vi "get_double.vi"(8 "error in (no error)":errorcluster, 11 "TrajectoryTS090820Circular2D in":refnum<class "TrajectoryTS090820Circular2D.lvclass">) -> (0 "error out":errorcluster, 2 "double":bool, 3 "TrajectoryTS090820Circular2D out":refnum<class "TrajectoryTS090820Circular2D.lvclass">)   [LabVIEW 2010, in "TrajectoryTS090820Circular2D.lvclass"]
uses:
  TrajectoryTS090820Circular2D.lvclass
  TrajectoryTS090820Circular2D.lvclass/TrajectoryTS090820Circular2D.ctl
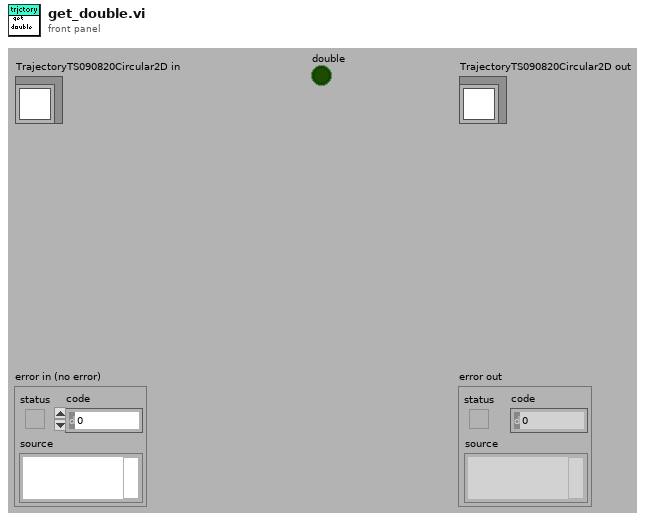
[diagram p1: front panel]
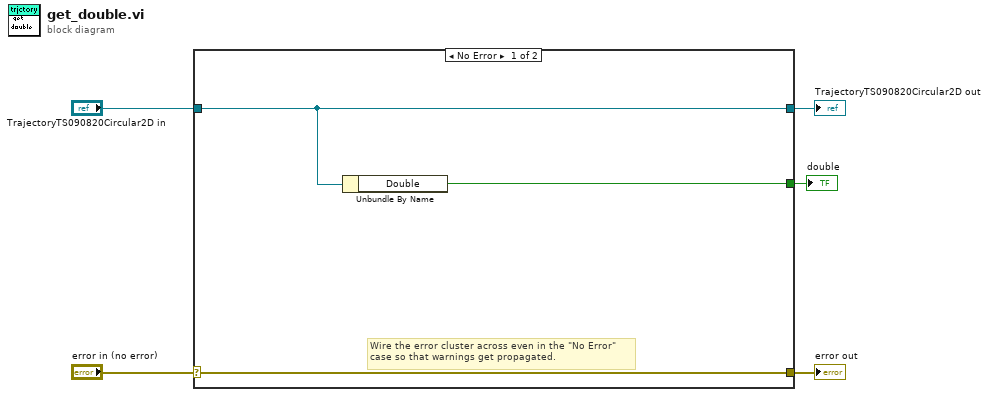
[diagram p0: block diagram]
diagram:
  n1 = case shown="No Error" "error in (no error)" {
    selector: "error in (no error)" -> [w8 w10]
    tunnel: [w8 w10] -> w4
    tunnel: [w7 w9] -> w2
    tunnel: "TrajectoryTS090820Circular2D in" -> [w7 w9]
    tunnel: [w6 _] -> w1
    frame No Error {
      # "Wire the error cluster across even in the \"No Error\"\ncase so that warnings get propagated."
      n2 = Unbundle By Name(w7) -> ("Double"=w6:bool)
    }
    frame Error {
    }
  }
  "error out" <- w4
  "TrajectoryTS090820Circular2D out" <- w2
  "double" <- w1
